vi "input-frame-engine.vi"(8 "error in (no error)":errorcluster, 11 "dbc in":refnum<class "bFrameIO.lvclass">) -> (0 "error out":errorcluster, 3 "dbc out":refnum<class "bFrameIO.lvclass">)   [LabVIEW 2015, in "bFrameIO.lvclass"]
uses:
  bFrameIO.lvclass
  bFrameIO.lvclass/bFrameIO.ctl
  controls/input-states.ctl
  read-baud-rate.vi
  read-fi-cluster.vi
  read-device.vi
  wrt-fi-state.vi
  read-fi-state.vi
  Read-frameQ.vi
  <vilib>/xnet/xnet.llb/XNET Create Session (Frame Input Stream).vi
  <vilib>/xnet/xnet.llb/XNET Read (Frame CAN).vi
  <resource>/objmgr/xnet.rc
  class.can.table/bAPPdata.lvclass
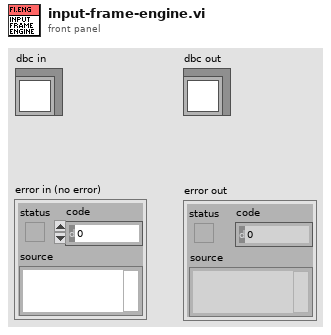
[diagram p1: front panel]
types:
  T1 = typedef "bFrameIO.lvclass/input-states.ctl" = enum16{"idle", "start", "run", "stop", "exit"}
  T2 = typedef "XNET Frame CAN.ctl" = cluster{"timestamp":timestamp, "payload":u8[], "identifier":u32, "type":T3, "extended?":bool, "echo?":bool}
  T3 = typedef "XNET Frame Type CAN.ctl" = u8
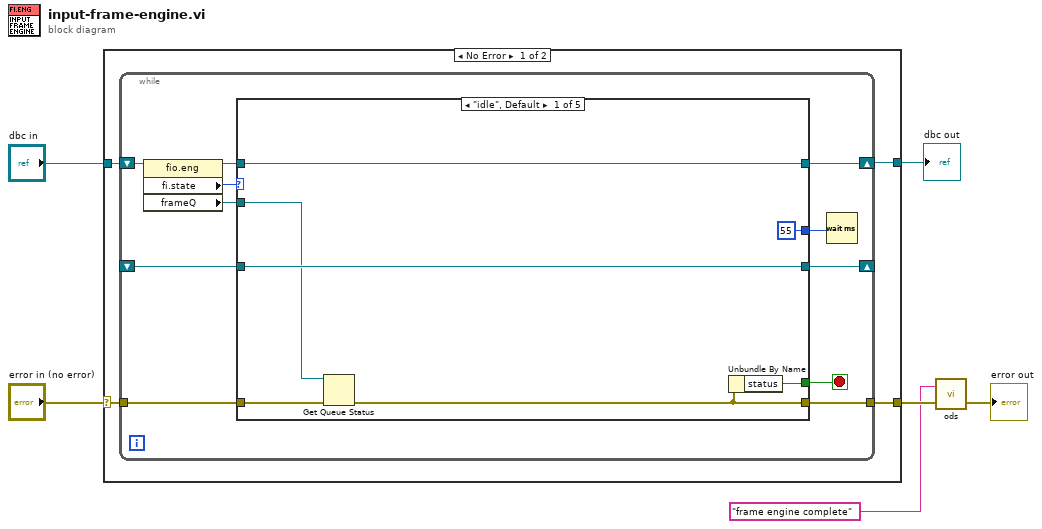
[diagram p0: block diagram]
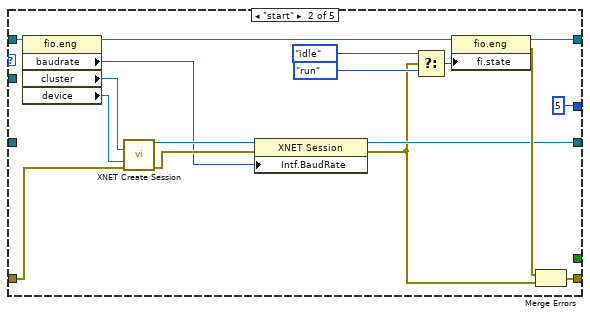
[diagram p2: hidden frame]
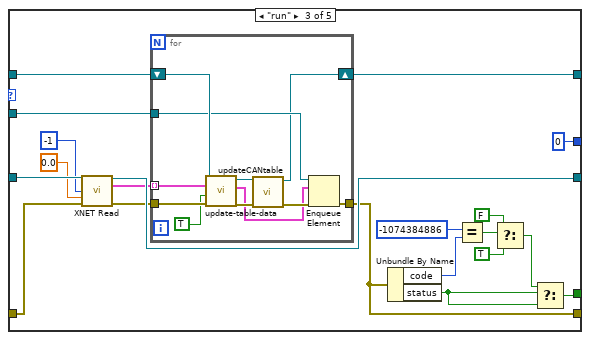
[diagram p3: hidden frame]
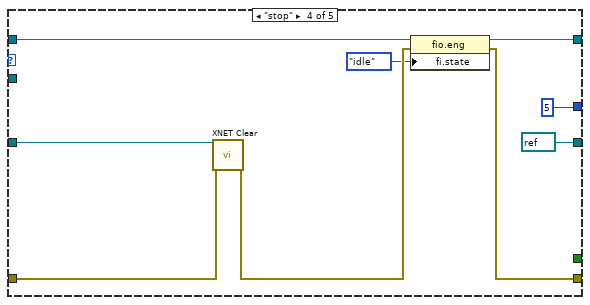
[diagram p4: hidden frame]
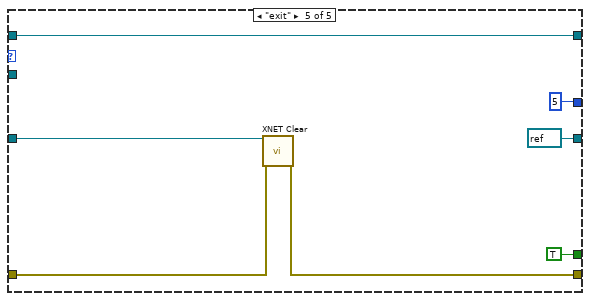
[diagram p5: hidden frame]
diagram:
  n1 = case shown="No Error" "error in (no error)" {
    selector: "error in (no error)" -> [w10 w94]
    tunnel: [w9 w94] -> w5
    tunnel: [w7 w93] -> w3
    tunnel: "dbc in" -> [w8 w93]
    frame No Error {
      n2 = while {
        tunnel: w10 -> [w12]
        tunnel: [w20] -> w9
        shift-right: [w18] -> w7
        shift-left: w8 -> [w21]
        shift-right: [w17] -> _
        shift-left: _ -> [w16]
        stop <- w15 stop-if-true
        n3 = property class="fio.eng"(reference=w21) -> (reference out=w19:refnum<class "bFrameIO.lvclass">, "fi.state"=w13:T1, "frameQ"=w11:refnum<queue>)  [unwired: 1 in, 1 out]
        n4 = case shown="\"idle\", Default" w13 {
          tunnel: w12 -> [w28 w43 w64 w81 w89]
          tunnel: [w23 w37 w50 w78 w88] -> w20
          tunnel: w19 -> [w27 w45 w61 w84 w92]
          tunnel: [w27 w42 w59 w80 w92] -> w18
          tunnel: [w26 w35 w62 refnum<k21> refnum ("session out") refnum<k21> refnum ("session out")] -> w17
          tunnel: w16 -> [w26 _ w65 w83 w91]
          tunnel: [w22 _ w55 _ TRUE] -> w15
          tunnel: [55 5 0 5 5] -> w14
          tunnel: w11 -> [w24 _ w46 _ _]
          frame "idle", Default {
            n5 = Get Queue Status(queue=w24, error in (no error)=w28) -> (error out=w23:errorcluster)  [unwired: 1 in, 7 out]
            n6 = Unbundle By Name(w23) -> ("status"=w22:bool)
          }
          frame "start" {
            n7 = property class="fio.eng"(reference=w45) -> (reference out=w36:refnum<class "bFrameIO.lvclass">, "baudrate"=w33:u32, "cluster"=w29:refnum<k21>, "device"=w30:refnum<k21>)  [unwired: 1 in, 1 out]
            n8 = call-poly <vilib>:"XNET Create Session.vi"("cluster (:memory:)"=w29, "interface"=w30, "error in (no error)"=w43) -> ("session out"=w44:refnum<k21>, "error out"=w34:errorcluster)  [unwired: 11 out]
            n9 = property class="XNET Session"(reference=w44, error in=w34, "Intf.BaudRate"=w33) -> (reference out=w35:refnum<k21>, error out=w32:errorcluster)
            n10 = Select(t=input-states."idle" ("fi.state"), s=w32, f=input-states."run") -> (s? t:f=w38:T1)
            n11 = property class="fio.eng"(reference=w36, "fi.state"=w38) -> (reference out=w42:refnum<class "bFrameIO.lvclass">, error out=w41:errorcluster)  [unwired: 1 in]
            n12 = Merge Errors(w41, w32) -> (w37:errorcluster)
          }
          frame "run" {
            n13 = call-poly <vilib>:"XNET Read.vi"("session in"=w65, "number to read (-1)"=-1, "timeout (0)"=0.0, "error in (no error)"=w64) -> ("session out"=w62:refnum<k21>, "data"=w47:T2[], "error out"=w60:errorcluster)  [unwired: 9 out]
            n14 = for {
              shift-right: [w67] -> w59
              shift-left: w61 -> [w76]
              tunnel: w60 -> [w75]
              tunnel: [w74] -> w50
              tunnel: w47 -> [w73] mode=indexing
              tunnel: w46 -> [w71]
              n15 = call "update-table-data.vi"("error in (no error)"=w75, "valid"=TRUE, "CAN frame"=w73, "CANtable in"=w76) -> ("error out"=w70:errorcluster, "CAN frame out"=w66:T2, "CANtable out"=w68:refnum<class "bFrameIO.lvclass">)  [unwired: 5 in]
              n16 = call "updateCANtable.vi"("error in (no error)"=w70, "CANtable.in"=w68) -> ("error out"=w69:errorcluster, "CANtable.out"=w67:refnum<class "bFrameIO.lvclass">)  [unwired: 8 in]
              n17 = Enqueue Element(queue=w71, element=w66, error in (no error)=w69) -> (error out=w74:errorcluster)  [unwired: 1 in, 2 out]
            }
            n18 = Unbundle By Name(w50) -> ("code"=w57:i32, "status"=w56:bool)
            n19 = Equal?(x=-1074384886, y=w57) -> (x = y?=w54:bool)
            n20 = Select(t=FALSE, s=w54, f=TRUE) -> (s? t:f=w51:bool)
            n21 = Select(t=w51, s=w56, f=w56) -> (s? t:f=w55:bool)
          }
          frame "stop" {
            n22 = call <vilib>:"XNET Clear.vi"("session in"=w83, "error in (no error)"=w81) -> ("error out"=w85:errorcluster)  [unwired: 13 in]
            n23 = property class="fio.eng"(reference=w84, error in=w85, "fi.state"=input-states."idle") -> (reference out=w80:refnum<class "bFrameIO.lvclass">, error out=w78:errorcluster)
          }
          frame "exit" {
            n24 = call <vilib>:"XNET Clear.vi"("session in"=w91, "error in (no error)"=w89) -> ("error out"=w88:errorcluster)  [unwired: 13 in]
          }
        }
        n25 = Wait (ms)(milliseconds to wait=w14) -> ()  [unwired: 1 out]
      }
    }
    frame Error {
    }
  }
  "dbc out" <- w3
  n26 = call "ods.vi"("error in (no error)"=w5, "str"="frame engine complete") -> ("error out"=→"error out":errorcluster)  [unwired: 1 in]
